vi "Read.vi"(8 "error in (no error)":errorcluster, 11 "Test Type B in":refnum<class "Test Type B.lvclass">) -> (0 "error out":errorcluster, 3 "Test Type B out":refnum<class "Test Type B.lvclass">)   [LabVIEW 2020, in "Test Type B.lvclass"]
uses:
  Test Type B.lvclass
  Test Type B.lvclass/Test Type B.ctl
panel:
  out "Value":dbl
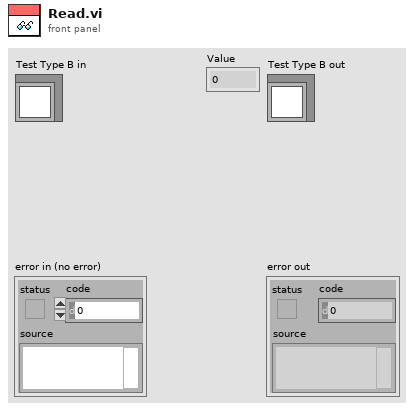
[diagram p1: front panel]
types:
  T1 = typedef "Test Type B.lvclass/Ref Data.ctl" = cluster{"Value":dbl}
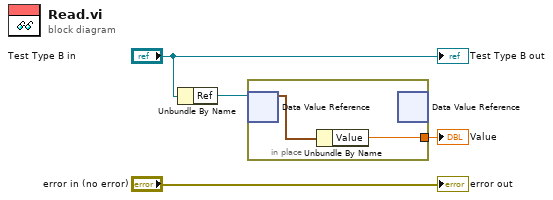
[diagram p0: block diagram]
diagram:
  n1 = Unbundle By Name("Test Type B in") -> ("Ref"=w3:refnum<data-value>)
  n2 = in-place {
    in-place-border: [w5] -> w1
    n3 = in-place-dvr #1(w3) -> (w6:T1)  [unwired: 1 out]
    n4 = Unbundle By Name(w6) -> ("Value"=w5:dbl)
    n5 = in-place-dvr #1() -> ()  [unwired: 1 in, 2 out]
  }
  "Value" <- w1
  "error out" <- "error in (no error)"
  "Test Type B out" <- "Test Type B in"
